vi "Measurement UI.vi"() -> ()   [LabVIEW 2024, in "Dynamic Signal Acquisition (Interactive) UI.lvlib"]
uses:
  Dynamic Signal Acquisition (Interactive) UI.lvlib
  <vilib>/Addons/_XControls/Waveforms with Cursors/Waveforms with Cursors.xctl
  <vilib>/addons/_XControls/Spectrum with Cursors/Spectrum with Cursors.xctl
  <vilib>/addons/_NISVFA/_Shared subVIs/Data Objects/Data/Data.lvclass
  SFPDAQ Configuration.ctl
  SFPDAQmx Channel Info.ctl
  <vilib>/addons/_NISVFA/_Shared subVIs/Data Objects/Y (DBL)/Y (N Ch).lvclass/Y (N Ch).ctl
  <vilib>/addons/_NISVFA/_Shared subVIs/Data Objects/Data/Data.lvclass/Data.ctl
  <vilib>/addons/_NISVFA/_Shared subVIs/Data Objects/Y (DBL)/SV Convert Spectra to Data Object.vi
  <vilib>/addons/_NISVFA/_Shared subVIs/Common/sv_Get NI Property Name String.vi
  <vilib>/addons/_NISVFA/_Shared subVIs/Data Objects/Data/Write Data Attributes.vi
  <vilib>/addons/_NISVFA/_Shared subVIs/Data Objects/subVIs/Set Channel Count.vi
  <vilib>/addons/_NISVFA/_Shared subVIs/Data Objects/Data/Read Data Attributes.vi
  <vilib>/addons/_NISVFA/_Shared subVIs/Data Objects/Y (DBL)/Y (N Ch).lvclass
  C:/Program Files/NI/LVAddons/nisvt/1/vi.lib/addons/_NISVFA/_Shared subVIs/Data Objects/Data/Data.lvclass
  <vilib>/addons/_NISVFA/_Shared subVIs/Data Objects/Y (DBL)/Write Channels Array.vi
  <vilib>/addons/_NISVFA/_Shared subVIs/Spectrum Info/sv_Convert Spectrum Info to Variant Attributes.vi
panel:
  out "packed waveforms":dbl[][](array[numeric])
  out "Waveforms":waveform(dbl)[](xcontrol)
  out "spectra info":string[][](array[string])
  out "packed spectra":dbl[][](array[numeric])
  out "Spectra":refnum<class "Data.lvclass">(xcontrol)
  out "measurements":bool
  out "DAQ trigger":u32
  out "DAQ channels":u32
  out "status":bool
  out "Trigger":u16(ring)
  out "Acquisition":u16(ring)
  out "Configuration":u16(ring)=1 caption="Task"
  in  "configure task":bool caption="Configure..."
  in  "DAQmx configuration json":string caption="DAQmx Configuration"
  in  "overlap":dbl=50.0 caption="Overlap" min=0.0 max=90.0 step=5.0 format="%#_g %"
  in  "window":u32(ring)=1 caption="Window" items=["None "=0, "Hanning"=1, "Flat Top"=6, "7 Term B-Harris"=8]
  out "averages":dbl caption="Averages Completed" format="%#_16f"
  out "averages completed":dbl caption="Averages Completed" format="%#_16f"
  in  "number of averages":dbl=10.0 caption="Number of Averages" min=1.0 max=1000.0 step=1.0
  in  "averaging mode":u32(ring) caption="Averaging Mode" items=["No averaging", "Vector averaging", "RMS averaging", "Peak hold"]
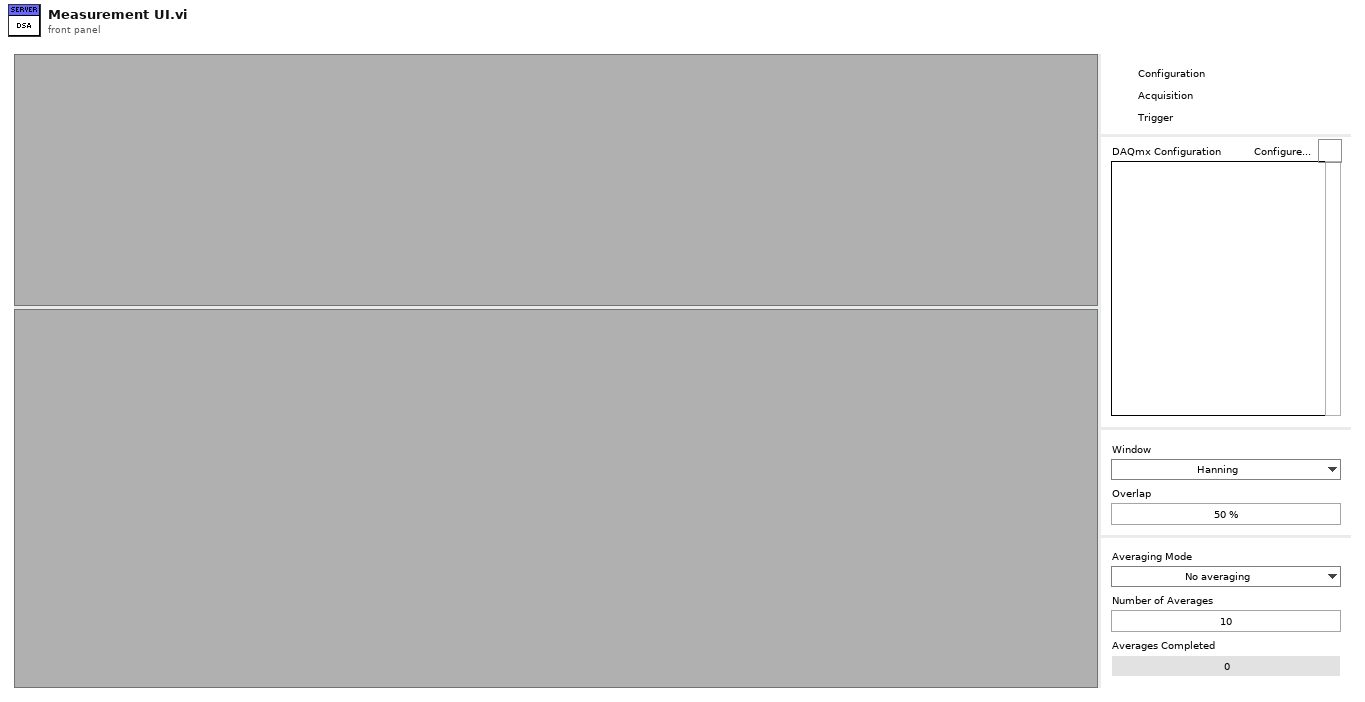
[diagram p1: front panel]
types:
  T1 = typedef "Dynamic Signal Acquisition (Interactive) UI.lvlib/SFPDAQ Configuration.ctl" = cluster{"Run Mode":u16, "Sample Rate (Hz)":dbl, "Block Size":i32, "Channel Table":T2[], "Trigger Type":u16, "Trigger Channel":string, "Level":dbl, "Pretrigger":i32, "Hysteresis":dbl, "Slope":enum16{"Falling", "Rising"}}
  T2 = typedef "Dynamic Signal Acquisition (Interactive) UI.lvlib/SFPDAQmx Channel Info.ctl" = cluster{"DAQmx Channel":tag, "Channel Type":u16, "Max":dbl, "Sensitivity":dbl, "Coupling":enum16{"AC", "DC"}, "input terminal configuration":i32, "excitation":enum16{"Off", "Min", "Max"}}
  T3 = enum8{"Enabled", "Disabled", "Disabled and Grayed Out"}
  T4 = typedef "LVRectTypeDef.ctl" = cluster{"Left":i16, "Top":i16, "Right":i16, "Bottom":i16}
  T5 = typedef "LVBoundsTypeDef.ctl" = cluster{"Width":u32, "Height":u32}
  T6 = typedef "LVPositionTypeDef.ctl" = cluster{"Left":i32, "Top":i32}
  T7 = typedef "SV_DAQmx.lvlib/Verification Status.ctl" = bool
  T8 = typedef "svc_Spectrum Info.ctl" = cluster{"channel name":string, "description":string, "x-axis units":T9, "spectral info":cluster{"spectrum type":T10, "linear/dB":enum16{"linear", "dB"}, "window":u16, "window size":i32, "FFT size":i32}, "engineering units":T11, "custom label":string, "dB reference [EU]":dbl, "peak units":enum16{"rms", "peak", "peak-peak"}, "weighting filter":T12, "spectral density?":bool, "unit label":string, "spectrum skewed?":bool, "complimentary spectrum units":T13}
  T9 = typedef "svc_X-Axis Units.ctl" = u16
  T10 = typedef "svc_Spectrum Type.ctl" = enum16{"FFT Spectrum [complex]", "Amplitude [Magnitude]", "Power [Magnitude^2]", "Cross Spectrum [complex]", "Frequency Response [Complex]"}
  T11 = typedef "svc_Engineering Units Text Ring.ctl" = u16
  T12 = typedef "svc_Weighting Filter Text Ring.ctl" = u16
  T13 = typedef "svc_Complimentary Spectrum Units.ctl" = enum16{"none", "radians", "degrees", "cycles", "imaginary"}
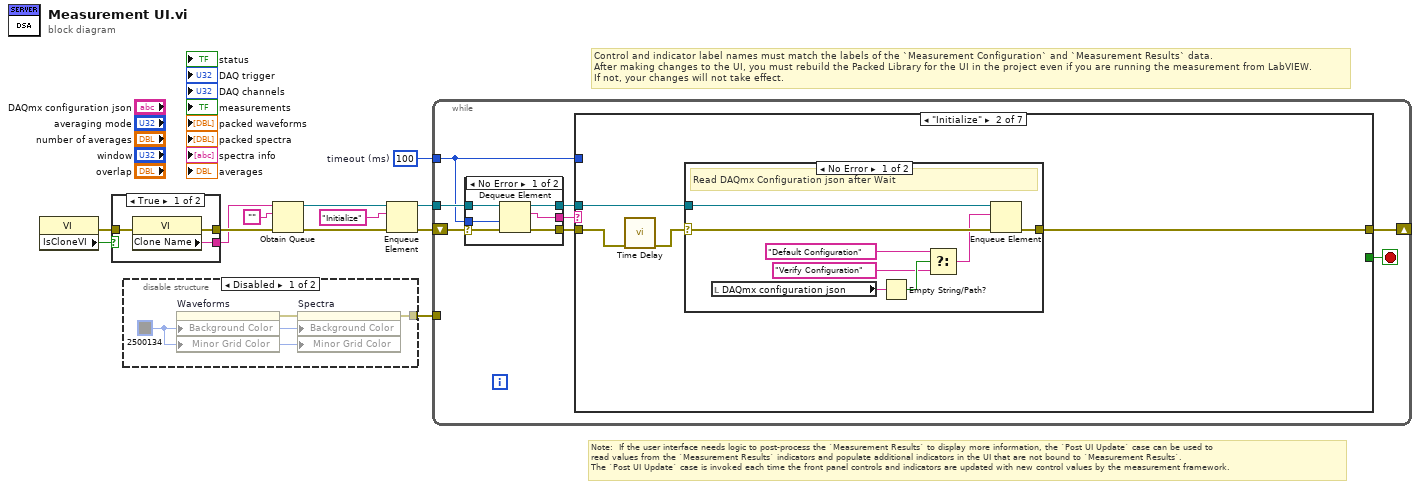
[diagram p0: block diagram]
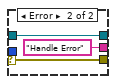
[diagram p2: hidden frame]
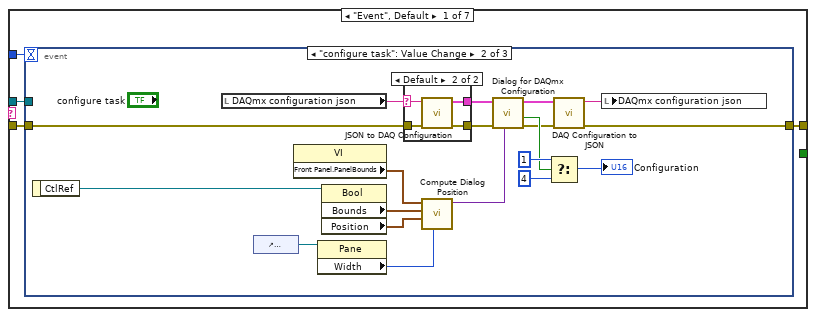
[diagram p3: hidden frame]
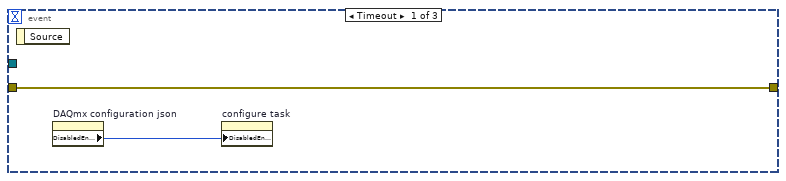
[diagram p4: hidden frame]
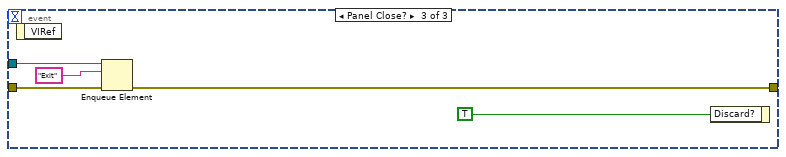
[diagram p6: hidden frame]
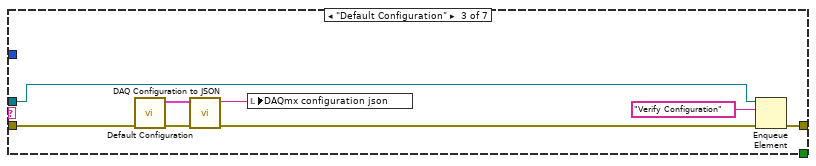
[diagram p8: hidden frame]
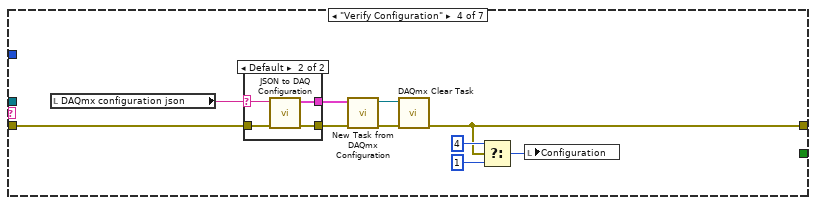
[diagram p9: hidden frame]
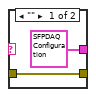
[diagram p10: hidden frame]
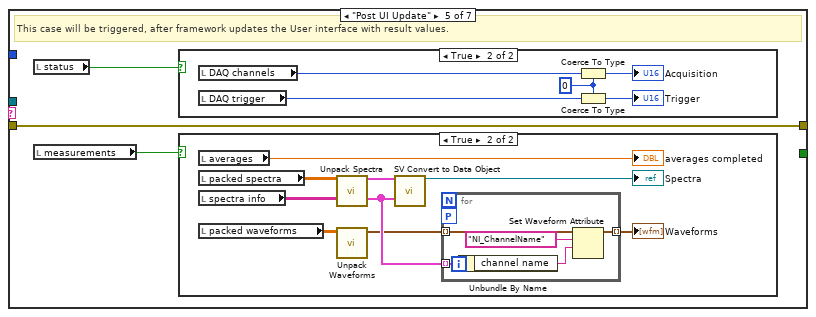
[diagram p11: hidden frame]
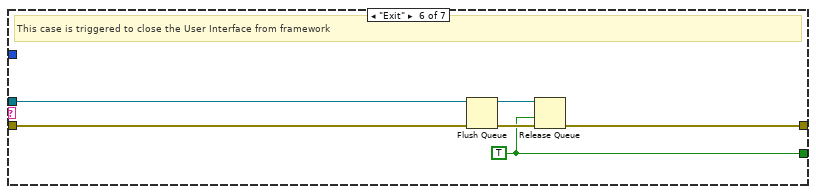
[diagram p14: hidden frame]
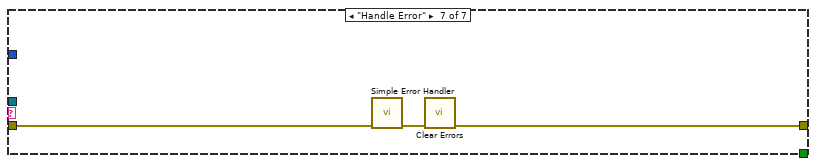
[diagram p15: hidden frame]
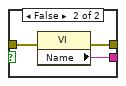
[diagram p17: hidden frame]
diagram:
  w2 = 100  # timeout (ms)
  # "Note:  If the user interface needs logic to post-process the `Measurement Results` to display more information, the `Post UI Update` case can be used to \nread values from the `Measurement Results` indicators and populate additional indicators in the UI that are not bound to `Measurement Results`. \nThe `Post UI Update` case is invoked each time the front panel controls and indicators are updated with new control values by the measurement framework."
  # "Control and indicator label names must match the labels of the `Measurement Configuration` and `Measurement Results` data. \nAfter making changes to the UI, you must rebuild the Packed Library for the UI in the project even if you are running the measurement from LabVIEW. \nIf not, your changes will not take effect."
  n1 = property class="VI"() -> (error out=w3:errorcluster, "IsCloneVI"=w4:bool)  [unwired: 2 in, 1 out]
  n2 = case shown="True" w4 {
    tunnel: [w15 w18] -> w12
    tunnel: [w14 w17] -> w11
    tunnel: w3 -> [w13 w16]
    frame True {
      n3 = property class="VI"(error in=w13) -> (error out=w15:errorcluster, "Clone Name"=w14:string)  [unwired: 1 in, 1 out]
    }
    frame False {
      n4 = property class="VI"(error in=w16) -> (error out=w18:errorcluster, "Name"=w17:string)  [unwired: 1 in, 1 out]
    }
  }
  n5 = disable-structure shown="Disabled" {
    disable-tunnel: [w19 _] -> w1
    frame Disabled {
      w21 = u32 2500134
      n6 = property on="Waveforms" class="Waveforms with Cursors (strict)"("Background Color"=w21, "Minor Grid Color"=w21) -> (error out=w20:errorcluster)  [unwired: 2 in, 1 out]
      n7 = property on="Spectra" class="Spectrum with Cursors (strict)"(error in=w20, "Background Color"=w21, "Minor Grid Color"=w21) -> (error out=w19:errorcluster)  [unwired: 1 in, 1 out]
    }
    frame Enabled {
    }
  }
  n8 = Obtain Queue(name (unnamed)=w11, element data type="", error in (no error)=w12) -> (queue out=w8:refnum<queue>, error out=w10:errorcluster)  [unwired: 2 in, 1 out]
  n9 = Enqueue Element(queue=w8, element="Initialize", error in (no error)=w10) -> (queue out=w7:refnum<queue>, error out=w9:errorcluster)  [unwired: 1 in, 1 out]
  n10 = while {
    shift-right: [w25] -> _
    shift-left: w9 -> [w29]
    tunnel: w7 -> [w27]
    tunnel: w2 -> [w23]
    tunnel: w1 -> [_]
    stop <- w24 stop-if-true
    n11 = case shown="No Error" w29 {
      selector: w29 -> [w35 w38]
      tunnel: [w34 w38] -> w28
      tunnel: w27 -> [w33 w37]
      tunnel: [w32 w37] -> w26
      tunnel: [w31 "Handle Error"] -> w22
      tunnel: w23 -> [w30 _]
      frame No Error {
        n12 = Dequeue Element(queue=w33, timeout in ms (-1)=w30, error in (no error)=w35) -> (queue out=w32:refnum<queue>, element=w31:string, error out=w34:errorcluster)  [unwired: 1 out]
      }
      frame Error {
      }
    }
    n13 = case shown="\"Initialize\"" w22 {
      tunnel: w28 -> [w41 w78 w90 w101 w113 w138 w141]
      tunnel: w26 -> [w40 w75 w91 _ _ w137 _]
      tunnel: [w42 w76 w92 w96 w113 w133 w140] -> w25
      tunnel: [_ _ _ _ _ w134 _] -> w24
      tunnel: w23 -> [w39 _ _ _ _ _ _]
      frame "Event", Default {
        n14 = event shown="[1] \"configure task\": Value Change" {
          selector: _ -> [_ _ _]
          dyn-events: _ -> [_ _ _]
          timeout: w39 -> [_ _ _]
          tunnel: [w44 w61 w72] -> w42
          tunnel: w41 -> [w44 w62 w73]
          tunnel: w40 -> [_ _ w71]
          event Timeout {
            n15 = event-data() -> ()  [unwired: 1 in, 1 out]
            n16 = property on="DAQmx configuration json" class="Str"() -> ("DisabledEnum"=w43:T3)  [unwired: 2 in, 2 out]
            n17 = property on="configure task" class="Bool"("DisabledEnum"=w43) -> ()  [unwired: 2 in, 2 out]
          }
          event "configure task": Value Change {
            n18 = event-data() -> ("CtlRef"=w63:refnum<vi>)  [unwired: 1 in]
            n19 = local read "DAQmx configuration json"() -> (w59:string)
            n20 = control-ref of="Waveforms Pane"() -> (w45:refnum<vi>)
            n21 = property class="VI"() -> ("Front Panel.PanelBounds"=w50:T4)  [unwired: 2 in, 2 out]
            n22 = property class="Pane"(reference=w45) -> ("Width"=w51:u32)  [unwired: 1 in, 2 out]
            n23 = property class="Bool"(reference=w63) -> ("Bounds"=w49:T5, "Position"=w48:T6)  [unwired: 1 in, 2 out]
            n24 = case shown="Default" w59 {
              selector: w59 -> [_ w69]
              tunnel: w62 -> [w65 w68]
              tunnel: [w65 w67] -> w57
              tunnel: [T1 {"Run Mode"=0, "Sample Rate (Hz)"=51200.0, "Block Size"=5120, "Channel Table"=[{"DAQmx Channel"="Dev1/ai0", "Channel Type"=0, "Max"=5.0, "Sensitivity"=1000.0, "Coupling"=enum."DC", "input terminal configuration"=-1, "excitation"=enum."Off"}], "Trigger Type"=0, "Trigger Channel"="", "Level"=0.0, "Pretrigger"=20, "Hysteresis"=0.0, "Slope"=enum."Rising"} ("DAQmx Configuration") w66] -> w58
              frame "" {
              }
              frame Default {
                n25 = call "JSON to DAQ Configuration.vi"("error in"=w68, "flattened JSON configuration"=w69) -> ("error out"=w67:errorcluster, "DAQmx Configuration"=w66:T1)  [unwired: 8 in]
              }
            }
            n26 = call "Compute Dialog Position.vi"("graph pane width"=w51, "launch button position"=w48, "launch button bounds"=w49, "front panel bounds"=w50) -> ("variant with position attribute"=w56:variant)  [unwired: 7 in]
            n27 = call "Dialog for DAQmx Configuration.vi"("Variant"=w56, "error in"=w57, "DAQmx config in"=w58) -> ("error out"=w46:errorcluster, "Task Verified"=w52:T7, "DAQmx config out"=w47:T1)  [unwired: 5 in, 1 out]
            n28 = Select(t=u16 1 ("Task"), s=w52, f=u16 4 ("Task")) -> (s? t:f=→"Configuration":u16)
            n29 = call "DAQ Configuration to JSON.vi"("error in"=w46, "DAQmx Configuration"=w47) -> ("error out"=w61:errorcluster, "flattened JSON configuration"=w60:string)  [unwired: 8 in]
            n30 = local write "DAQmx configuration json"(w60) -> ()
          }
          event Panel Close? {
            n31 = event-data() -> ()  [unwired: 1 in, 1 out]
            n32 = Enqueue Element(queue=w71, element="Exit", error in (no error)=w73) -> (error out=w72:errorcluster)  [unwired: 1 in, 2 out]
            n33 = event-data("Discard?"=TRUE) -> ()  [unwired: 1 in, 1 out]
          }
        }
      }
      frame "Initialize" {
        n34 = call "Time Delay"("error in (no error)"=w78) -> ("error out"=w77:errorcluster)  [unwired: 10 in]
        n35 = case shown="No Error" w77 {
          selector: w77 -> [w85 w87]
          tunnel: [w83 w87] -> w76
          tunnel: w75 -> [w84 _]
          frame No Error {
            # "Read DAQmx Configuration json after Wait"
            n36 = local read "DAQmx configuration json"() -> (w86:string)
            n37 = Empty String/Path?(string/path=w86) -> (empty?=w82:bool)
            n38 = Select(t="Default Configuration" ("element"), s=w82, f="Verify Configuration" ("element")) -> (s? t:f=w79:string)
            n39 = Enqueue Element(queue=w84, element=w79, error in (no error)=w85) -> (error out=w83:errorcluster)  [unwired: 1 in, 2 out]
          }
          frame Error {
          }
        }
      }
      frame "Default Configuration" {
        n40 = call "Default Configuration.vi"() -> ("DAQmx Configuration"=w89:T1)  [unwired: 11 in]
        n41 = call "DAQ Configuration to JSON.vi"("error in"=w90, "DAQmx Configuration"=w89) -> ("error out"=w93:errorcluster, "flattened JSON configuration"=w88:string)  [unwired: 8 in]
        n42 = local write "DAQmx configuration json"(w88) -> ()
        n43 = Enqueue Element(queue=w91, element="Verify Configuration", error in (no error)=w93) -> (error out=w92:errorcluster)  [unwired: 1 in, 2 out]
      }
      frame "Verify Configuration" {
        n44 = local read "DAQmx configuration json"() -> (w95:string)
        n45 = case shown="Default" w95 {
          selector: w95 -> [_ w110]
          tunnel: w101 -> [w106 w109]
          tunnel: [w106 w108] -> w100
          tunnel: [T1 {"Run Mode"=0, "Sample Rate (Hz)"=51200.0, "Block Size"=5120, "Channel Table"=[{"DAQmx Channel"="Dev1/ai0", "Channel Type"=0, "Max"=5.0, "Sensitivity"=1000.0, "Coupling"=enum."DC", "input terminal configuration"=-1, "excitation"=enum."Off"}], "Trigger Type"=0, "Trigger Channel"="", "Level"=0.0, "Pretrigger"=20, "Hysteresis"=0.0, "Slope"=enum."Rising"} ("DAQmx Configuration") w107] -> w99
          frame "" {
          }
          frame Default {
            n46 = call "JSON to DAQ Configuration.vi"("error in"=w109, "flattened JSON configuration"=w110) -> ("error out"=w108:errorcluster, "DAQmx Configuration"=w107:T1)  [unwired: 8 in]
          }
        }
        n47 = call "New Task from DAQmx Configuration.vi"("error in"=w100, "DAQmx Cfg"=w99) -> ("error out"=w98:errorcluster, "DAQmx task"=w97:refnum<k21>)  [unwired: 8 in]
        n48 = call <vilib>:"DAQmx Clear Task.vi"("task in"=w97, "error in"=w98) -> ("error out"=w96:errorcluster)  [unwired: 13 in]
        n49 = Select(t=u16 4 ("Task"), s=w96, f=u16 1 ("Task")) -> (s? t:f=w104:u16)
        n50 = local write "Configuration"(w104) -> ()
      }
      frame "Post UI Update" {
        # "This case will be triggered, after framework updates the User interface with result values."
        n51 = local read "status"() -> (w112:bool)
        n52 = local read "measurements"() -> (w111:bool)
        n53 = case shown="True" w112 {
          frame False {
          }
          frame True {
            w128 = u16 0 ("Acquisition")
            n54 = local read "DAQ channels"() -> (w132:u32)
            n55 = local read "DAQ trigger"() -> (w131:u32)
            n56 = Coerce To Type(0:w132, 1:w128) -> (2:→"Acquisition":u16)
            n57 = Coerce To Type(0:w131, 1:w128) -> (2:→"Trigger":u16)
          }
        }
        n58 = case shown="True" w111 {
          frame False {
          }
          frame True {
            n59 = local read "averages"() -> (→"averages completed":dbl)
            n60 = local read "packed spectra"() -> (w116:dbl[][])
            n61 = local read "spectra info"() -> (w115:string[][])
            n62 = local read "packed waveforms"() -> (w117:dbl[][])
            n63 = call "Unpack Spectra.vi"("packed spectra"=w116, "spectra info"=w115) -> ("spectra"=w122:cluster{"f0":dbl, "df":dbl, "magnitude":dbl[]}[], "spectrum info"=w120:T8[])  [unwired: 16 in]
            n64 = call "Unpack Waveforms.vi"("packed waveforms"=w117) -> ("waveforms"=w119:waveform(dbl)[])  [unwired: 10 in]
            n65 = call-poly <vilib>:"SV Convert to Data Object.vi"("spectra"=w122, "spectra info"=w120) -> ("Spectrum Data"=→"Spectra":refnum<class "Data.lvclass">)  [unwired: 16 in, 1 out]
            n66 = for {
              tunnel: [w126] -> w118 mode=indexing
              tunnel: w119 -> [w127] mode=indexing
              workers-P: _ -> [_]
              tunnel: w120 -> [w125] mode=indexing
              n67 = Unbundle By Name(w125) -> ("channel name"=w123:string)
              n68 = Set Waveform Attribute(5:w123, 6:"NI_ChannelName" ("name"), 7:w127) -> (3:w126:waveform(dbl))  [unwired: 1 in, 2 out]
            }
            "Waveforms" <- w118
          }
        }
      }
      frame "Exit" {
        w134 = TRUE ("force destroy? (F)")
        # "This case is triggered to close the User Interface from framework"
        n69 = Flush Queue(queue=w137, error in (no error)=w138) -> (queue out=w136:refnum<queue>, error out=w135:errorcluster)  [unwired: 1 out]
        n70 = Release Queue(queue=w136, force destroy? (F)=w134, error in (no error)=w135) -> (error out=w133:errorcluster)  [unwired: 2 out]
      }
      frame "Handle Error" {
        n71 = call <vilib>:"Simple Error Handler.vi"("error in (no error)"=w141) -> ("error out"=w139:errorcluster)  [unwired: 4 in, 4 out]
        n72 = call <vilib>:"Clear Errors.vi"("error in (no error)"=w139) -> ("error out"=w140:errorcluster)  [unwired: 5 in, 1 out]
      }
    }
  }
